vi "file - read-write - list of lines-V2.vi"(7 "read/write control":T1, 9 "header IN":string, 10 "list of lines IN":string[](array[string]), 11 "file path":path=path "/opt/new/Dropbox/shared_AkashAndreas/paper-CeCoIn5/dataset--changeT--12T--0deg--60deg--90deg/CeCoIn5_4th__129_(043)__C(f)_12T_0.255K_45deg_changeT_raw_.dat") -> (1 "header OUT":string, 2 "list of lines OUT":string[](array[string]), 3 "filename out":string)   [LabVIEW 2020]
uses:
  file -- read-write control.ctl
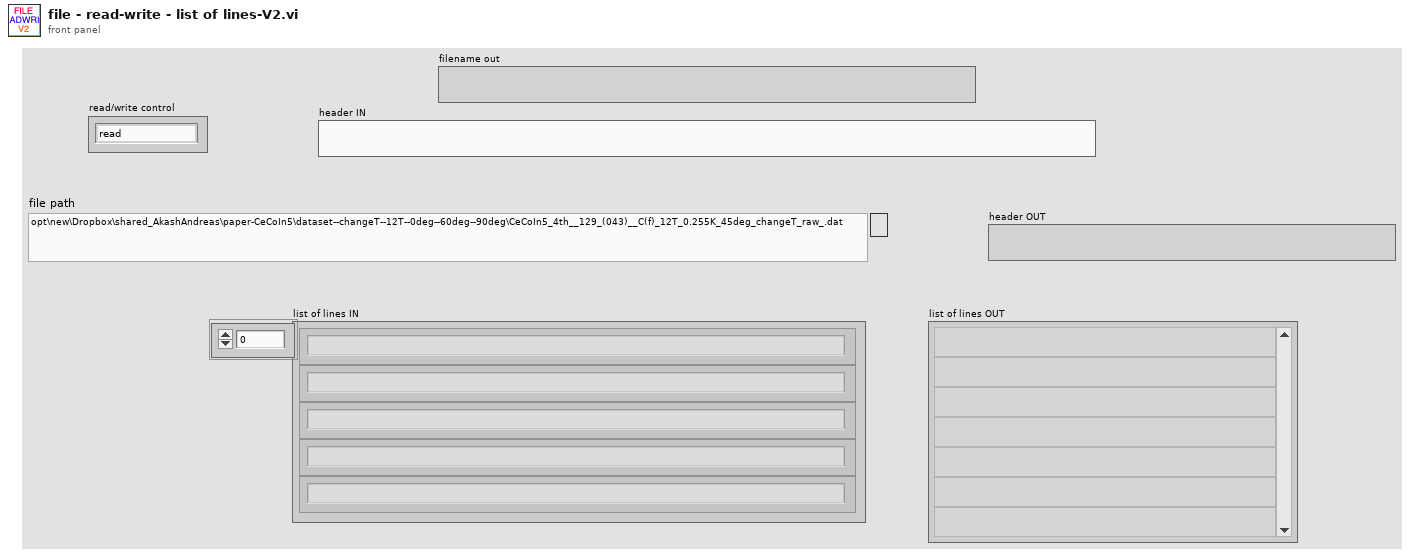
[diagram p1: front panel]
types:
  T1 = typedef "file -- read-write control.ctl" = enum16{"read", "write all", "append one line"}
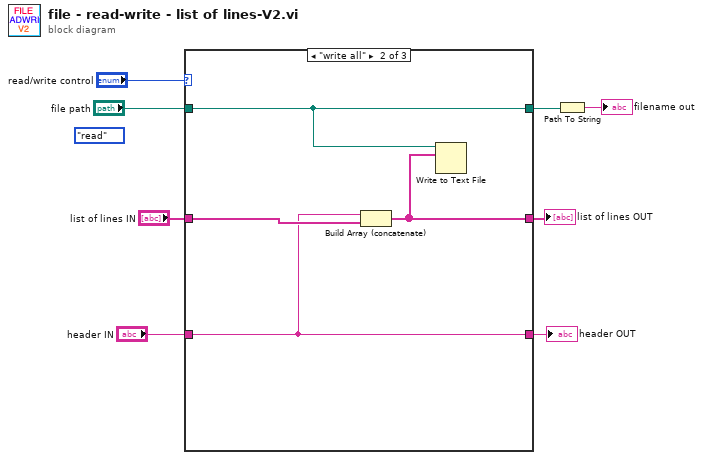
[diagram p0: block diagram]
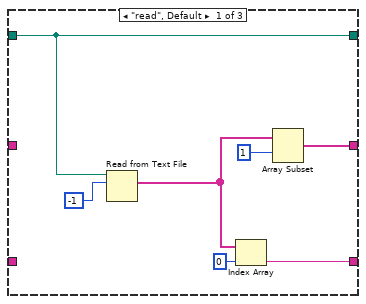
[diagram p2: hidden frame]
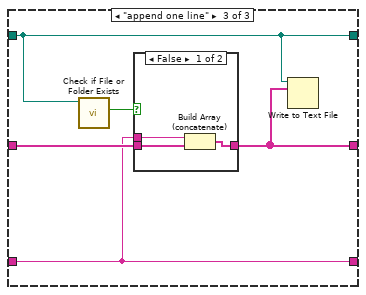
[diagram p3: hidden frame]
diagram:
  (unwired) file_--_read-write_control."read" ("read/write control")
  n1 = case shown="\"write all\"" "read/write control" {
    tunnel: "file path" -> [w9 w16 w20]
    tunnel: [w10 w17 w21] -> w8
    tunnel: [w13 w18 w22] -> w7
    tunnel: "header IN" -> [_ w18 w22]
    tunnel: "list of lines IN" -> [_ w19 w23]
    tunnel: [w9 w16 w20] -> w1
    frame "read", Default {
      n2 = Read from Text File(file (use dialog)=w9, count=-1) -> (text=w12:string[])  [unwired: 2 in, 3 out]
      n3 = Index Array(array=w12, index=0) -> (element=w13:string)
      n4 = Array Subset(array=w12, index=1 ("length")) -> (w10:string[])  [unwired: 1 in]
    }
    frame "write all" {
      n5 = Build Array (concatenate)(w18, w19) -> (w17:string[])
      n6 = Write to Text File(file (use dialog)=w16, text=w17) -> ()  [unwired: 2 in, 3 out]
    }
    frame "append one line" {
      n7 = call <vilib>:"Check if File or Folder Exists.vi"("path"=w20) -> ("file or folder exists?"=w24:bool)  [unwired: 8 in, 2 out]
      n8 = case shown="False" w24 {
        tunnel: w23 -> [w27 w28]
        tunnel: w22 -> [w26 _]
        tunnel: [w25 w28] -> w21
        frame False {
          n9 = Build Array (concatenate)(w26, w27) -> (w25:string[])
        }
        frame True {
        }
      }
      n10 = Write to Text File(file (use dialog)=w20, text=w21) -> ()  [unwired: 2 in, 3 out]
    }
  }
  "list of lines OUT" <- w8
  "header OUT" <- w7
  n11 = Path To String(path=w1) -> (string=→"filename out":string)
